vi "aimTest1553.vi"() -> ()   [LabVIEW 2020]
panel:
  out "Module Handle":u32
  out "Reset Information":T1 {"Sim Buffer Addr" format="%08x"; "Sim Buffer Size" format="%08x"; "Bus Mon Buffer Addr" format="%08x"; "Bus Mon Buffer Size" format="%08x"}
  out "Error Out":errorcluster {"code" format="%x"}
  in  "Module Number (0)":u32
  in  "Self test mode (none)":T2(ring)
  in  "Debug Flags (0x3000 0000)":T3={"Interrupt"=FALSE, "Initialization"=FALSE, "Module open"=FALSE, "Module close"=FALSE, "Module I/O"=FALSE, "Module recording"=FALSE, "Replay"=FALSE, "Mutex"=FALSE, "Parameter range check"=FALSE, "(internal use)"=FALSE, "Function call trace log"=FALSE, "Informational"=TRUE, "General errors"=TRUE, "Force error message box"=FALSE}
  in  "error in":errorcluster
  in  "Stream ID":u32=1
  # "Simulator Buffer"
  # "Size"
  # "Address"
  # "Bus Monitor Buffer"
  # "Size"
  # "Address"
  # "Force debug outputs related to:"
  # "log to file: aim_mil.log"
  # "e.g.: range check, etc."
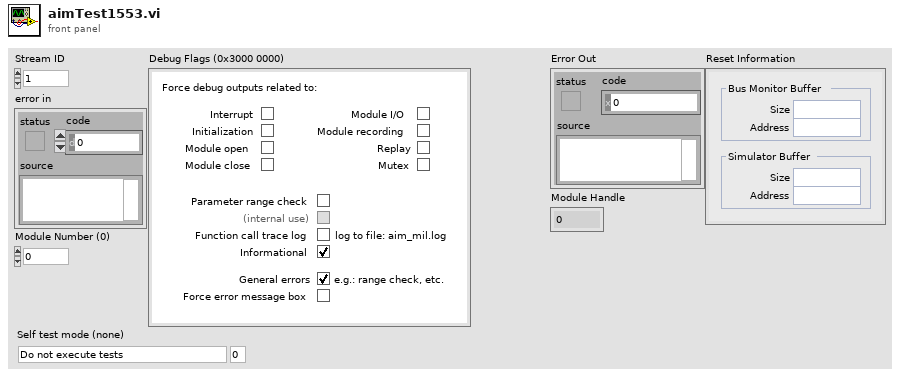
[diagram p1: front panel]
types:
  T1 = cluster{"Bus Mon Buffer Size":u8, "Sim Buffer Size":u8, "Bus Mon Buffer Addr":u32, "Sim Buffer Addr":u32}
  T2 = enum16{"Do not execute tests", "Execute all tests", "Board enable test", "Internal self-test", "Global RAM test for BIU control block", "Global RAM test for BIU BC/RT descriptor", "Global RAM test for BIU bus monitor", "Shared RAM test from 0x100000", "Shared RAM test for CMD area", "Shared RAM test for ACK area", "Transfer test", "Interrupt test", "DAC test for bus A", "DAC test for bus B", "Timing test"}
  T3 = cluster{"Interrupt":bool, "Initialization":bool, "Module open":bool, "Module close":bool, "Module I/O":bool, "Module recording":bool, "Replay":bool, "Mutex":bool, "Parameter range check":bool, "(internal use)":bool, "Function call trace log":bool, "Informational":bool, "General errors":bool, "Force error message box":bool}
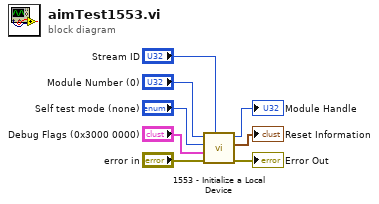
[diagram p0: block diagram]
diagram:
  n1 = call <instrlib>:"1553 - Initialize a Local Device.vi"("Stream ID"="Stream ID", "Error In"="error in", "Debug Flags (0x3000 0000)"="Debug Flags (0x3000 0000)", "Self test mode (none)"="Self test mode (none)", "Module Number (0)"="Module Number (0)") -> ("Error Out"=→"Error Out":errorcluster, "Reset Information"=→"Reset Information":T1, "Module Handle"=→"Module Handle":u32)  [unwired: 4 in]
